vi "DetectChange.vi"(11 "Variant":variant) -> (3 "Change?":bool)   [LabVIEW 2014]
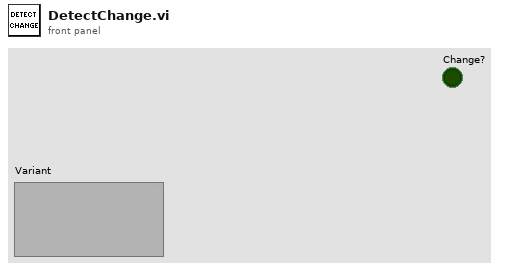
[diagram p1: front panel]
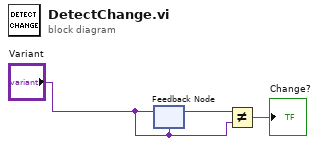
[diagram p0: block diagram]
diagram:
  n1 = feedback-in #1("Variant") -> ()
  n2 = feedback #1("Variant") -> (w3:variant)
  n3 = Not Equal?(x=w3, y="Variant") -> (x != y?=→"Change?":bool)
